vi "Do.vi"(8 "error in (no error)":errorcluster, 10 "Actor in":refnum<class "Actor.lvclass">, 11 "Measure [MSR] Msg":refnum<class "Measure [MSR] Msg.lvclass">) -> (0 "error out":errorcluster, 2 "Actor out":refnum<class "Actor.lvclass">)   [LabVIEW 2013, in "CS++DMM.lvlib" / "Measure [MSR] Msg.lvclass"]
doc: "This VI delivers the message to the actor by calling the appropriate method(s) on the actor."
uses:
  Measure [MSR] Msg.lvclass
  CS++DCPwr/CS++DCPwr.lvclass
  <vilib>/ActorFramework/Actor/Actor.lvclass
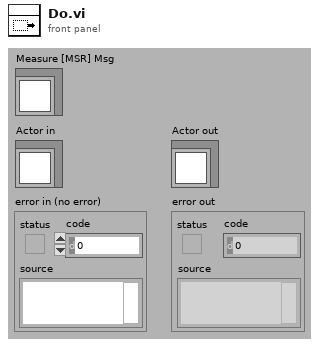
[diagram p1: front panel]
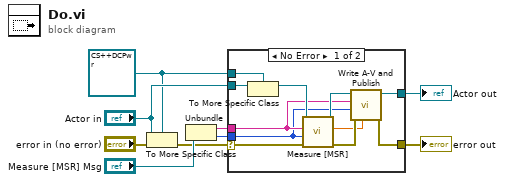
[diagram p0: block diagram]
diagram:
  w3 = refnum<class "CS++DCPwr.lvclass"> refnum ("Actor in")
  n1 = To More Specific Class(target class=w3, reference="Actor in", error in="error in (no error)") -> (error out=w7:errorcluster)  [unwired: 1 out]
  n2 = Unbundle("Measure [MSR] Msg") -> (w2:string, w1:i32)
  n3 = case shown="No Error" w7 {
    selector: w7 -> [w20 w22]
    tunnel: [w13 w22] -> w6
    tunnel: [w15 w21] -> w5
    tunnel: "Actor in" -> [w19 w21]
    tunnel: w3 -> [w18 _]
    tunnel: w2 -> [w12 _]
    tunnel: w1 -> [w11 _]
    frame No Error {
      n4 = To More Specific Class(target class=w18, reference=w19) -> (specific class reference=w17:refnum<class "CS++DCPwr.lvclass">)  [unwired: 1 in, 1 out]
      n5 = call-dynamic "Measure [MSR].vi"("error in (no error)"=w20, "measurement type (voltage)"=w11, "channel name (\"CHANNEL1\")"=w12, "Cs++DCPwr in"=w17) -> ("error out"=w14:errorcluster, "measurement"=w10:dbl, "CS++DCPwr out"=w16:refnum<class "CS++DCPwr.lvclass">)  [unwired: 5 in]
      n6 = call "Write A-V and Publish.vi"("measurement"=w10, "error in (no error)"=w14, "measurement type (voltage)"=w11, "channel name (\"CHANNEL1\")"=w12, "CS++DCPwr in"=w16) -> ("error out"=w13:errorcluster, "CS++DCPwr out"=w15:refnum<class "CS++DCPwr.lvclass">)  [unwired: 5 in]
    }
    frame Error {
    }
  }
  "error out" <- w6
  "Actor out" <- w5
